vi "clearpath_process.vi"(0 "ClearpathComm":T1) -> ()   [LabVIEW 2010, in "clearpath_interface.lvlib"]
doc: "Constantly processes incoming and outgoing serial data. Transmits anything in the transmit queue (blocking transmits on acknowledgements), receives and parses incoming data, places valid data into the received data queue"
uses:
  clearpath_interface.lvlib
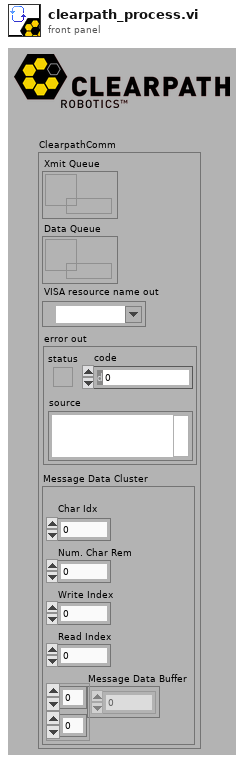
[diagram p1: front panel]
types:
  T1 = cluster{"Xmit Queue":refnum<queue>, "Data Queue":refnum<queue>, "VISA resource name out":refnum<visa-resource-name>, "error out":errorcluster, "Message Data Cluster":cluster{"\nChar Idx":u8, "Num. Char Rem":u8, "Write Index":u8, "Read Index":u8, "Message Data Buffer":u8[][]}}
  T2 = cluster{"\nChar Idx":u8, "Num. Char Rem":u8, "Write Index":u8, "Read Index":u8, "Message Data Buffer":u8[][]}
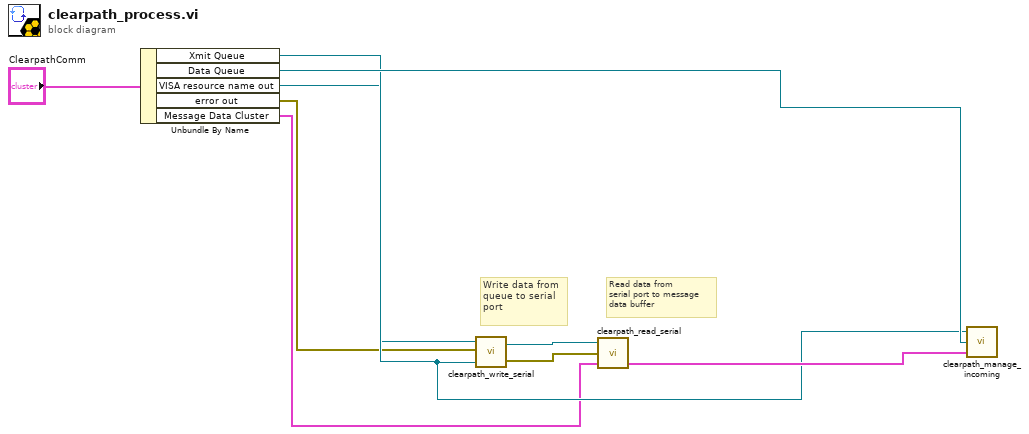
[diagram p0: block diagram]
diagram:
  # "Read data from\nserial port to message\ndata buffer"
  # "Write data from\nqueue to serial \nport"
  n1 = Unbundle By Name("ClearpathComm") -> ("Xmit Queue"=w5:refnum<queue>, "Data Queue"=w6:refnum<queue>, "VISA resource name out"=w1:refnum<visa-resource-name>, "error out"=w2:errorcluster, "Message Data Cluster"=w3:T2)
  n2 = call "clearpath_write_serial.vi"("queue in"=w5, "error in"=w2, "VISA resource name in"=w1) -> ("error out"=w8:errorcluster, "VISA resource name out"=w7:refnum<visa-resource-name>)
  n3 = call "clearpath_read_serial.vi"("Cluster In"=w3, "error in"=w8, "VISA resource name in"=w7) -> ("Cluster Out"=w9:T2)  [unwired: 2 out]
  n4 = call "clearpath_manage_incoming.vi"("Message Data Cluster In"=w9, "Data Queue"=w6, "Xmit Queue"=w5) -> ()  [unwired: 1 out]
